vi "Add Component Dependencies.vi"(8 "error in (no error)":errorcluster, 11 "Device Item Ref in":T1 format="%.0x") -> (0 "error out":errorcluster, 2 "component names":string[](array[string]), 3 "Device Ref out":T1 format="%.0x")   [LabVIEW 2017, in "DSF System Explorer.lvlib"]
uses:
  DSF System Explorer.lvlib
  <vilib>/NI Veristand/Custom Device API/Custom Device Item Ref.ctl
  <vilib>/NI Veristand/Custom Device API/Set Item Property (Path).vi
  <vilib>/NI Veristand/Custom Device API/Custom Device API.lvlib
  Shared/DSF Shared.lvlib
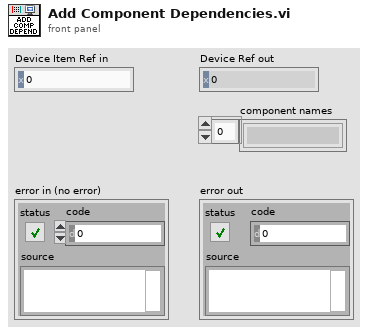
[diagram p1: front panel]
types:
  T1 = typedef "Custom Device API.lvlib/Custom Device Item Ref.ctl" = u64
  T2 = typedef "Custom Device API.lvlib/Custom Device Target Type.ctl" = enum16{"PharLap", "VxWorks", "Windows", "Linux_32_ARM", "Linux_x64"}
  T3 = typedef "Custom Device API.lvlib/Custom Device File Dependency.ctl" = cluster{"Source":T4, "RT Destination":path, "ForceDownload?":bool, "SupportedTarget":T6, "Version":string}
  T4 = typedef "Custom Device API.lvlib/Path Specification.ctl" = cluster{"Path":path, "Type":T5}
  T5 = typedef "Custom Device API.lvlib/Path Type.ctl" = enum16{"Absolute", "To Base", "To Common Data Dir", "To Application Data Dir"}
  T6 = typedef "Custom Device API.lvlib/Custom Device Supported Target.ctl" = enum16{"All", "PharLap", "VxWorks", "Windows", "Linux_32_ARM", "Linux_x64", "PharLap & Windows", "PharLap & VxWorks", "VxWorks & Windows"}
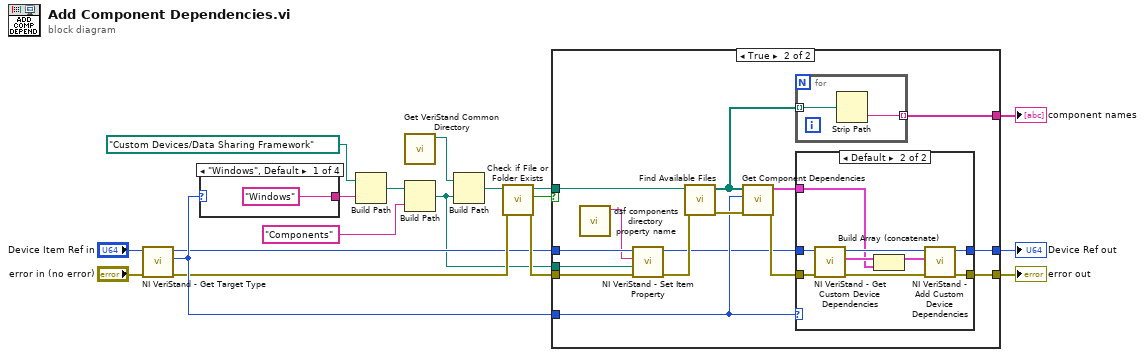
[diagram p0: block diagram]
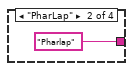
[diagram p4: hidden frame]
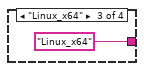
[diagram p5: hidden frame]
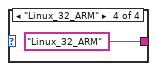
[diagram p6: hidden frame]
diagram:
  n1 = call <vilib>:"NI VeriStand - Get Target Type.vi"("error in (no error)"="error in (no error)", "Item Ref in"="Device Item Ref in") -> ("error out"=w8:errorcluster, "Target Type"=w12:T2, "Item Ref out"=w6:T1)  [unwired: 7 in]
  n2 = case shown="\"Windows\", Default" w12 {
    tunnel: ["Windows" "Pharlap" "Linux_x64" "Linux_32_ARM"] -> w14
    frame "Windows", Default {
    }
    frame "PharLap" {
    }
    frame "Linux_x64" {
    }
    frame "Linux_32_ARM" {
    }
  }
  n3 = Build Path(base path=path "Custom Devices/Data Sharing Framework", name or relative path=w14) -> (appended path=w15:path)
  n4 = call "Get VeriStand Common Directory.vi"() -> ("common directory"=w17:path)  [unwired: 11 in]
  n5 = Build Path(base path=w15, name or relative path="Components") -> (appended path=w1:path)
  n6 = Build Path(base path=w17, name or relative path=w1) -> (appended path=w2:path)
  n7 = call <vilib>:"Check if File or Folder Exists.vi"("error in (no error)"=w8, "path"=w2) -> ("error out"=w7:errorcluster, "file or folder exists?"=w5:bool, "dup path"=w9:path)  [unwired: 7 in]
  n8 = case shown="True" w5 {
    tunnel: [w23 w39] -> w18
    tunnel: [w24 w38] -> w4
    tunnel: [_ w33] -> w13
    tunnel: w6 -> [w23 w32]
    tunnel: w12 -> [_ w31]
    tunnel: w9 -> [_ w27]
    tunnel: w7 -> [w24 w26]
    tunnel: w1 -> [_ w25]
    frame False {
    }
    frame True {
      n9 = call "dsf components directory property name.vi"() -> ("components directory property name"=w28:string)  [unwired: 11 in]
      n10 = call-poly <vilib>:"NI VeriStand - Set Item Property.vi"("error in (no error)"=w26, "Value"=w25, "Property Name"=w28, "Item Ref in"=w32) -> ("error out"=w30:errorcluster, "Item Ref out"=w29:T1)  [unwired: 5 in, 1 out]
      n11 = call "Find Available Files.vi"("error in (no error)"=w30, "components directory"=w27) -> ("error out"=w35:errorcluster, "paths"=w34:path[])  [unwired: 8 in]
      n12 = call "Get Component Dependencies.vi"("error in (no error)"=w35, "Target Type"=w31, "component paths"=w34) -> ("error out"=w37:errorcluster, "component dependencies"=w36:T3[])  [unwired: 7 in]
      n13 = for {
        tunnel: w34 -> [w41] mode=indexing
        tunnel: [w40] -> w33 mode=indexing
        n14 = Strip Path(path=w41) -> (name=w40:string)  [unwired: 1 out]
      }
      n15 = case shown="Default" w31 {
        tunnel: w36 -> [_ w45]
        tunnel: w37 -> [w43 w51]
        tunnel: w29 -> [w42 w52]
        tunnel: [w43 w46] -> w38
        tunnel: [w42 w44] -> w39
        frame "Windows" {
          # "Don't add dependencies for Windows."
        }
        frame Default {
          n16 = call <vilib>:"NI VeriStand - Get Custom Device Dependencies.vi"("error in (no error)"=w51, "Device Ref in"=w52) -> ("error out"=w49:errorcluster, "Dependencies"=w50:T3[], "Device Ref out"=w47:T1)  [unwired: 7 in]
          n17 = Build Array (concatenate)(w50, w45) -> (w48:T3[])
          n18 = call <vilib>:"NI VeriStand - Add Custom Device Dependencies.vi"("error in (no error)"=w49, "Dependencies"=w48, "Device Ref in"=w47) -> ("error out"=w46:errorcluster, "Device Ref out"=w44:T1)  [unwired: 7 in]
        }
      }
    }
  }
  "Device Ref out" <- w18
  "error out" <- w4
  "component names" <- w13
